vi "Image roto-translation top level.vi"(0 "ROI to crop (pixels)":T2={"Xmax"=2147483647, "Ymax"=2147483647, "Xmin"=0, "Ymin"=0}, 1 "Theta range (deg)":T1={"theta max (deg)"=180.0, "theta min (deg)"=-180.0}, 2 "Iters":i32=15, 3 "Apply scaling":bool, 4 "Apply rotation":bool=TRUE, 5 "Apply Tx":bool=TRUE, 6 "Test image file path":path=path "C:/Users/Paul Nathan/Desktop/Building test pictures/Building_pos_9.jpg", 7 "Apply Ty":bool=TRUE, 8 "Reference image file path":path=path "C:/Users/Paul Nathan/Desktop/Building test pictures/Building_pos_1.jpg", 9 "Keep proc. img":bool, 11 "Auto ROI (for rot.)":bool) -> (14 "Scale factor":dbl, 15 "Rotation (deg)":dbl, 16 "Tx (pixels)":dbl, 17 "Ty (pixels)":dbl, 18 "Processed test img path":path, 19 "Error Out":errorcluster)   [LabVIEW 2015]
uses:
  Typedefs/ROI bounds.ctl
  Typedefs/Theta range.ctl
panel:
  out "Iter":i32
  out "Image out":T3(plugin-control)
  # "Paul Nathan 10/06/2015, \n07/12/2015"
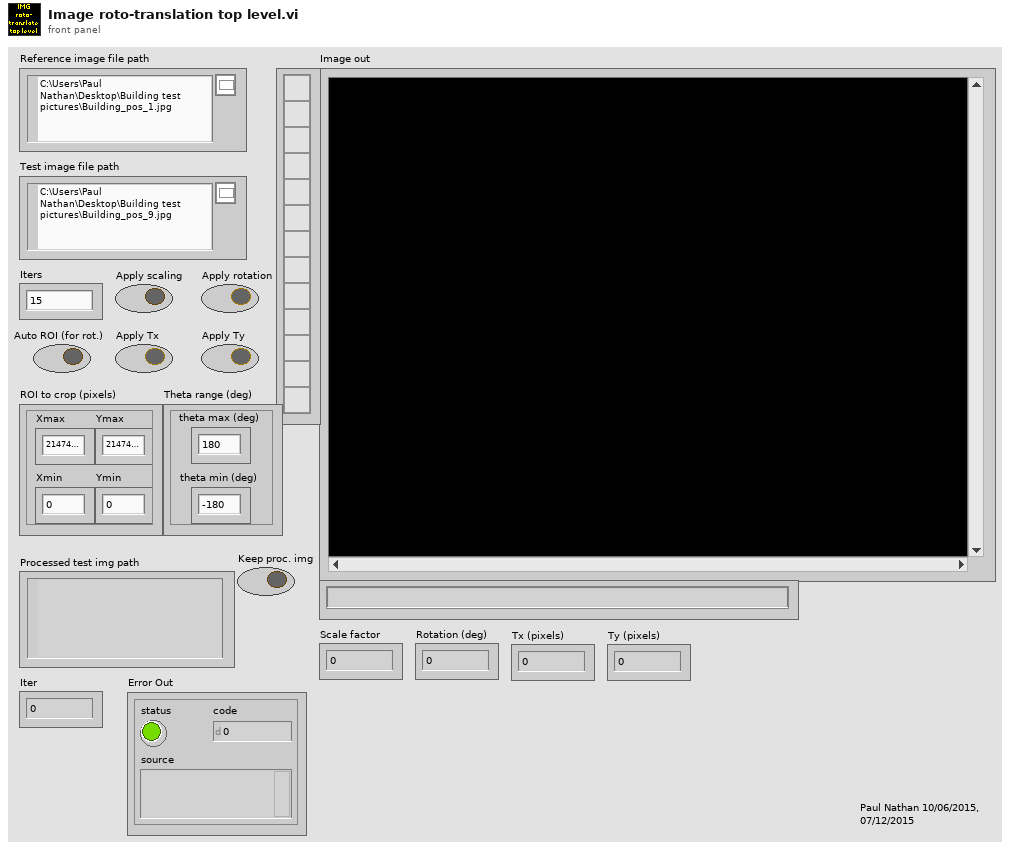
[diagram p1: front panel]
types:
  T1 = typedef "Theta range.ctl" = cluster{"theta max (deg)":dbl, "theta min (deg)":dbl}
  T2 = typedef "ROI bounds.ctl" = cluster{"Xmax":i32, "Ymax":i32, "Xmin":i32, "Ymin":i32}
  T3 = typedef "IMAQ Image.ctl" = refnum<image>
  T4 = typedef "Image Type" = u32
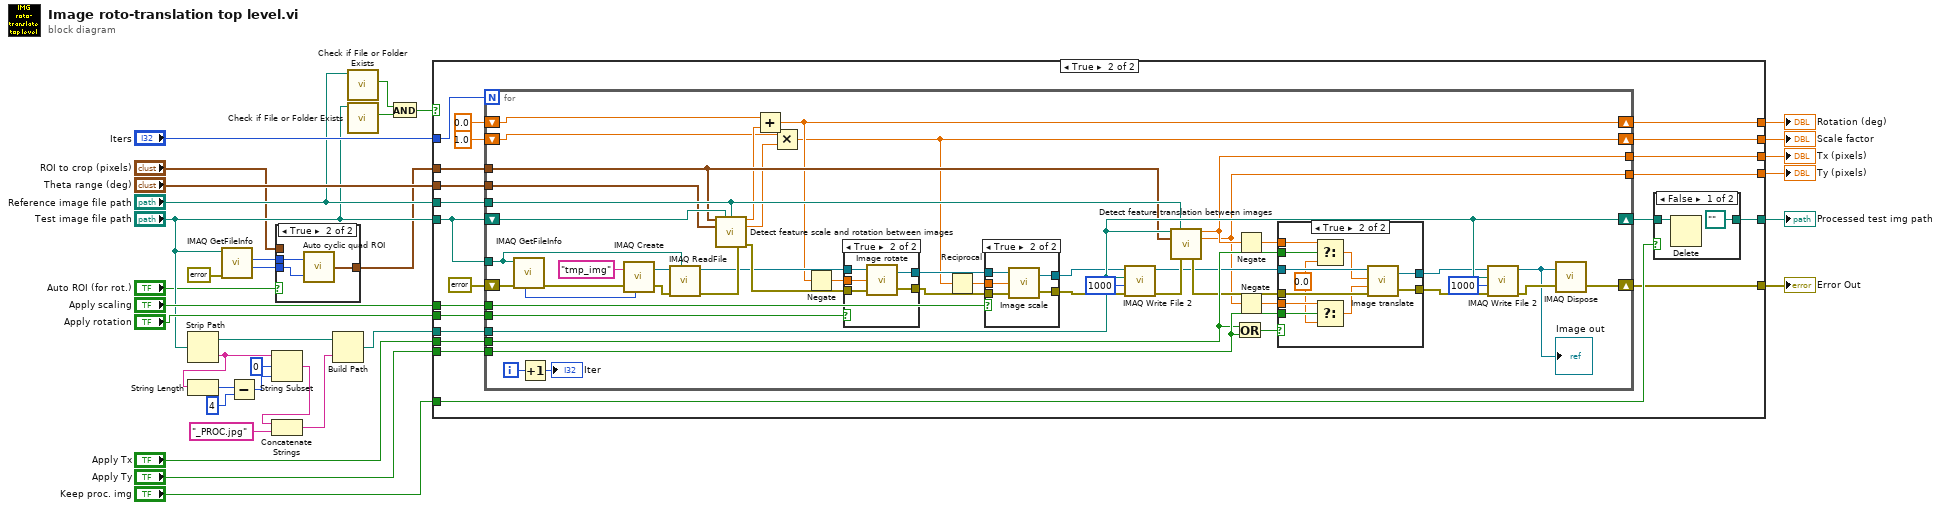
[diagram p0: block diagram]
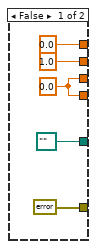
[diagram p3: hidden frame]
diagram:
  n1 = Strip Path(path="Test image file path") -> (stripped path=w26:path, name=w32:string)
  n2 = String Length(string=w32) -> (length=w31:i32)
  n3 = call "IMAQ GetFileInfo"("error in (no error)"=errorcluster {"status"=FALSE, "code"=0, "source"=""}, "File Path"="Test image file path") -> ("Y Resolution"=w3:i32, "X Resolution"=w4:i32)  [unwired: 3 in, 5 out]
  n4 = Subtract(x=w31, y=4) -> (x-y=w25:i32)
  n5 = String Subset(string=w32, offset (0)=0, length (rest)=w25) -> (substring=w29:string)
  n6 = Concatenate Strings(w29, "_PROC.jpg" ("name or relative path")) -> (w27:string)
  n7 = case shown="True" "Auto ROI (for rot.)" {
    tunnel: [w35 w36] -> w5
    tunnel: w4 -> [_ w38]
    tunnel: w3 -> [_ w37]
    tunnel: "ROI to crop (pixels)" -> [w35 _]
    frame False {
    }
    frame True {
      n8 = call "Auto cyclic quad ROI.vi"("img_H"=w37, "img_W"=w38) -> ("ROI to crop (pixels)"=w36:T2)
    }
  }
  n9 = Build Path(base path=w26, name or relative path=w27) -> (appended path=w33:path)
  n10 = call <vilib>:"Check if File or Folder Exists.vi"("path"="Reference image file path") -> ("file or folder exists?"=w15:bool)  [unwired: 8 in, 2 out]
  n11 = call <vilib>:"Check if File or Folder Exists.vi"("path"="Test image file path") -> ("file or folder exists?"=w16:bool)  [unwired: 8 in, 2 out]
  n12 = And(x=w15, y=w16) -> (x .and. y?=w14:bool)
  n13 = case shown="True" w14 {
    tunnel: "Reference image file path" -> [_ w64]
    tunnel: "Iters" -> [_ w63]
    tunnel: w33 -> [_ w62]
    tunnel: [0.0 ("Rotation (deg)") w44] -> w9
    tunnel: [w42 w49] -> w11
    tunnel: "Test image file path" -> [_ w52]
    tunnel: [1.0 ("Rotation (deg)") w45] -> w8
    tunnel: "Apply scaling" -> [_ w61]
    tunnel: "Apply rotation" -> [_ w60]
    tunnel: w5 -> [_ w59]
    tunnel: "Apply Tx" -> [_ w58]
    tunnel: "Apply Ty" -> [_ w57]
    tunnel: "Theta range (deg)" -> [_ w56]
    tunnel: [path "" ("Test image file path") w53] -> w18
    tunnel: [errorcluster {"status"=FALSE, "code"=0, "source"=""} ("error in (no error)") w51] -> w12
    tunnel: "Keep proc. img" -> [_ w55]
    tunnel: [w42 w48] -> w10
    frame False {
      w42 = 0.0 ("dx (pix)")
    }
    frame True {
      n14 = for {
        N: w63 -> [_]
        tunnel: w64 -> [w92]
        shift-right: [w112] -> w54
        shift-left: w52 -> [w91]
        tunnel: w62 -> [w112]
        shift-right: [w79] -> w51
        shift-left: errorcluster {"status"=FALSE, "code"=0, "source"=""} ("error in (no error)") -> [w81]
        tunnel: w61 -> [w99]
        tunnel: w60 -> [w96]
        tunnel: w59 -> [w90]
        tunnel: w58 -> [w93]
        tunnel: w57 -> [w94]
        tunnel: w56 -> [w89]
        tunnel: w52 -> [w78]
        shift-right: [w70] -> w44
        shift-left: 0.0 ("Rotation (deg)") -> [w72]
        shift-right: [w67] -> w45
        shift-left: 1.0 ("Rotation (deg)") -> [w68]
        tunnel: [w74] -> w49
        tunnel: [w73] -> w48
        i -> [w98]
        n15 = call "IMAQ GetFileInfo"("error in (no error)"=w81, "File Path"=w78) -> ("error out"=w87:errorcluster, "Image Type"=w88:T4)  [unwired: 3 in, 5 out]
        n16 = Increment(x=w98) -> (x+1=→"Iter":i32)
        n17 = call "IMAQ Create"("Image Name"="tmp_img", "Image Type"=w88, "error in (no error)"=w87) -> ("New Image"=w85:T3, "error out"=w86:errorcluster)  [unwired: 2 in]
        n18 = call "IMAQ ReadFile"("File Path"=w78, "error in (no error)"=w86, "Image"=w85) -> ("error out"=w83:errorcluster, "Image Out"=w82:T3)  [unwired: 4 in, 3 out]
        n19 = call "Detect feature scale and rotation between images.vi"("ROI to crop (pixels)"=w90, "Test image file path"=w91, "Reference image file path"=w92, "Theta range (deg)"=w89, "Error In"=w83) -> ("Rotation (deg)"=w71:dbl, "Scale factor"=w69:dbl, "Error out"=w109:errorcluster)  [unwired: 6 in, 2 out]
        n20 = Add(x=w72, y=w71) -> (x+y=w70:dbl)
        n21 = Multiply(x=w68, y=w69) -> (x*y=w67:dbl)
        n22 = Negate(x=w70) -> (-x=w108:dbl)
        n23 = case shown="True" w96 {
          tunnel: w82 -> [w114 w119]
          tunnel: w109 -> [w113 w118]
          tunnel: w108 -> [_ w117]
          tunnel: [w114 w116] -> w103
          tunnel: [w113 w115] -> w102
          frame False {
          }
          frame True {
            n24 = call "Image rotate.vi"("Error in"=w118, "Rotation angle, ccw+ (deg)"=w117, "Image in"=w119) -> ("Error Out"=w115:errorcluster, "Image Out"=w116:T3)
          }
        }
        n25 = Reciprocal(x=w67) -> (1/x=w100:dbl)
        n26 = case shown="True" w99 {
          tunnel: w103 -> [w121 w126]
          tunnel: [w121 w125] -> w66
          tunnel: w102 -> [w120 w124]
          tunnel: [w120 w123] -> w101
          tunnel: w100 -> [_ w122]
          frame False {
          }
          frame True {
            n27 = call "Image scale.vi"("Error in"=w124, "Scale factor"=w122, "Image in"=w126) -> ("Error Out"=w123:errorcluster, "Image Out"=w125:T3)
          }
        }
        n28 = call-poly "IMAQ Write File 2"("error in (no error)"=w101, "Image Quality"=u32 1000, "File Path"=w112, "Image"=w66) -> ("error out"=w76:errorcluster, "Image Out (duplicate)"=w75:T3)  [unwired: 6 in]
        n29 = call "Detect feature translation between images.vi"("Test image file path"=w112, "Reference image file path"=w92, "ROI to crop (pixels)"=w90, "Error In"=w76) -> ("dx (pix)"=w74:dbl, "dy (pix)"=w73:dbl, "Error out"=w77:errorcluster)  [unwired: 7 in, 2 out]
        n30 = Or(x=w93, y=w94) -> (x .or. y?=w95:bool)
        n31 = Negate(x=w74) -> (-x=w105:dbl)
        n32 = Negate(x=w73) -> (-x=w104:dbl)
        n33 = case shown="True" w95 {
          tunnel: w75 -> [w128 w139]
          tunnel: w77 -> [w127 w138]
          tunnel: [w128 w137] -> w107
          tunnel: [w127 w136] -> w106
          tunnel: w105 -> [_ w135]
          tunnel: w104 -> [_ w133]
          tunnel: w94 -> [_ w131]
          tunnel: w93 -> [_ w130]
          frame False {
          }
          frame True {
            w129 = 0.0 ("f")
            n34 = Select(t=w135, s=w130, f=w129) -> (s? t:f=w134:dbl)
            n35 = Select(t=w133, s=w131, f=w129) -> (s? t:f=w132:dbl)
            n36 = call "Image translate.vi"("Error in"=w138, "Ty (pix)"=w132, "Tx (pix)"=w134, "Image in"=w139) -> ("Error Out"=w136:errorcluster, "Image Out"=w137:T3)
          }
        }
        n37 = call-poly "IMAQ Write File 2"("error in (no error)"=w106, "Image Quality"=u32 1000, "File Path"=w112, "Image"=w107) -> ("error out"=w80:errorcluster, "Image Out (duplicate)"=w65:T3)  [unwired: 6 in]
        "Image out" <- w65
        n38 = call "IMAQ Dispose"("Image"=w65, "error in (no error)"=w80) -> ("error out"=w79:errorcluster)  [unwired: 4 in]
      }
      n39 = case shown="False" w55 {
        tunnel: w54 -> [w140 w142]
        tunnel: [path "" ("Test image file path") w142] -> w53
        frame False {
          n40 = Delete(path (use dialog)=w140) -> ()  [unwired: 4 in, 3 out]
        }
        frame True {
        }
      }
    }
  }
  "Processed test img path" <- w18
  "Error Out" <- w12
  "Tx (pixels)" <- w11
  "Ty (pixels)" <- w10
  "Rotation (deg)" <- w9
  "Scale factor" <- w8
